vi "Close.vi"(8 "error in":errorcluster, 11 "Cfg Dev in":refnum<class "Vaisala.lvclass">) -> (0 "error out":errorcluster, 3 "Cfg Dev out":refnum<class "Vaisala.lvclass">)   [LabVIEW 2015, in "Vaisala.lvclass"]
uses:
  Vaisala.lvclass
  Reusable/Session APIs/Text Communication/Text Device Session.lvclass
  Vaisala.lvclass/Vaisala.ctl
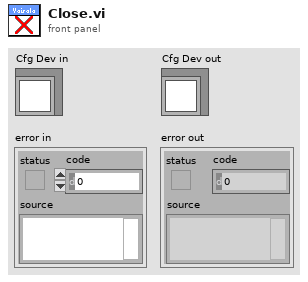
[diagram p1: front panel]
types:
  T1 = typedef "Session - Root.lvclass/Session Handle.ctl" = refnum<data-value>
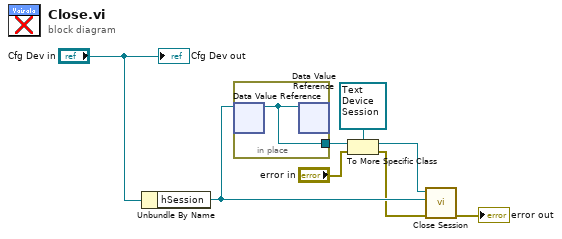
[diagram p0: block diagram]
diagram:
  n1 = Unbundle By Name("Cfg Dev in") -> ("hSession"=w8:T1)
  n2 = in-place {
    in-place-border: [w9] -> w7
    n3 = in-place-dvr #1(w8) -> (w9:refnum<class "Session - Root.lvclass">)  [unwired: 1 out]
    n4 = in-place-dvr #1(w9) -> ()  [unwired: 2 out]
  }
  n5 = To More Specific Class(target class=refnum<class "Text Device Session.lvclass"> refnum ("Text Session"), reference=w7, error in="error in") -> (specific class reference=w5:refnum<class "Text Device Session.lvclass">, error out=w2:errorcluster)
  n6 = call-dynamic "Close Session.vi"("error in"=w2, "Session In"=w8, "Text Session"=w5) -> ("error out"=→"error out":errorcluster)  [unwired: 7 in, 1 out]
  "Cfg Dev out" <- "Cfg Dev in"
